vi "Power Supply_Create.vi"(0 "reference in":refnum<class "Power Supply.lvclass">, 5 "error in (no error)":errorcluster) -> (14 "reference out":refnum<class "Power Supply.lvclass">, 19 "error out":errorcluster)   [LabVIEW 2017, in "Power Supply.lvclass"]
uses:
  Power Supply.lvclass
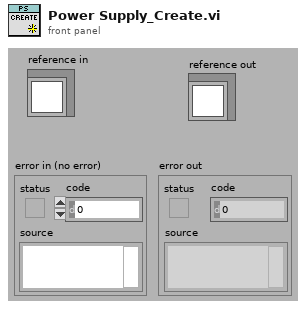
[diagram p1: front panel]
types:
  T1 = typedef "Power Supply.lvclass/ObjectAttributes.ctl" = cluster{"Power Supply Chain VISA Session":refnum<visa-resource-name>, "Power Supply Chain Address":i16, "Power Supply Open/Close Status":bool, "Power Supply Voltage Setting":dbl, "Power Supply Current Setting":dbl, "Power Supply Voltage Reading":dbl, "Power Supply Current Reading":dbl, "Power Supply Status":T2, "Power Supply Error":T3, "Fault Register":u8, "Power Supply Error":bool}
  T2 = typedef "Power Supply.lvclass/Power Supply Status.ctl" = enum16{"Closed", "Open"}
  T3 = typedef "Power Supply.lvclass/Power Supply Error.ctl" = enum16{"None", "Read Error"}
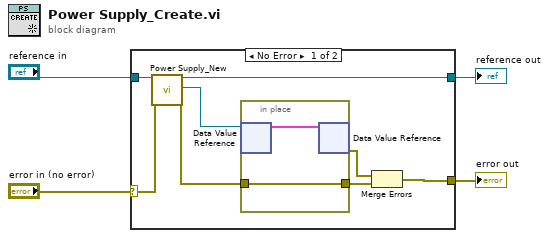
[diagram p0: block diagram]
diagram:
  n1 = case shown="No Error" "error in (no error)" {
    selector: "error in (no error)" -> [w11 w16]
    tunnel: [w8 w16] -> w3
    tunnel: "reference in" -> [w12 w15]
    tunnel: [w10 w15] -> w1
    frame No Error {
      n2 = call "Power Supply_New.vi"("reference in"=w12, "error in (no error)"=w11) -> ("reference out"=w10:refnum<class "Power Supply.lvclass">, "DVRRefOut"=w7:refnum<data-value>, "error out"=w6:errorcluster)  [unwired: 14 in, 1 out]
      n3 = in-place {
        in-place-border: w6 -> [w14]
        in-place-border: [w14] -> w5
        n4 = in-place-dvr #1(w7) -> (w13:T1)  [unwired: 1 out]
        n5 = in-place-dvr #1(w13) -> (w9:errorcluster)  [unwired: 1 out]
      }
      n6 = Merge Errors(w9, w5) -> (w8:errorcluster)
    }
    frame Error {
    }
  }
  "error out" <- w3
  "reference out" <- w1
